vi "Actor Core.vi"(8 "error in":errorcluster, 11 "Measure Object in":refnum<class "LabJack Recorder.lvclass">) -> (0 "error out":errorcluster, 3 "Actor out":refnum<class "Actor.lvclass">)   [LabVIEW 2021, in "LabJack Recorder.lvclass"]
doc: "(<B>Filename</B>: Actor Framework.lvlib:Actor.lvclass:Actor Core.vi)\n\nReceives messages to the actor, reacts to them, and initiates any error handling that may shut the actor down.\n\nDescendant classes may override this VI to append parallel tasks for the actor to complete while it handles messages. Overrides use the Call Parent Method node."
uses:
  LabJack Recorder.lvclass
  <vilib>/ActorFramework/Actor/Actor.lvclass
  NHMFL_Core/Libraries/Instruments/LabJack/LabJack Configuration.ctl
  Continuous Recorder Actor/Continuous Recorder Actor.lvclass
panel:
  in  "Configuration":T1={"Scale"=-443.074, "Offset"=532.969, "AIN Range"=0, "Positive channel #"=0, "Negativ channel #"=15} {"AIN Range" items=["LJ_rgBIP10V", "LJ_rgBIP1V", "LJ_rgBIPP1V", "LJ_rgBIPP01V"]}
  out "Name":string
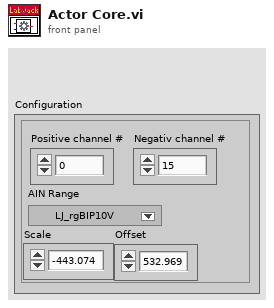
[diagram p1: front panel]
types:
  T1 = typedef "LabJack Configuration.ctl" = cluster{"Scale":dbl, "Offset":dbl, "AIN Range":u16, "Positive channel #":i32, "Negativ channel #":i32}
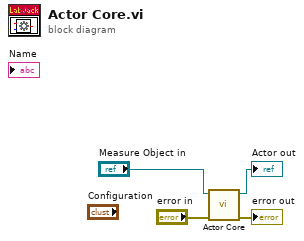
[diagram p0: block diagram]
diagram:
  n1 = call-parent "Actor Core.vi"("error in"="error in", "Measure Object in"="Measure Object in") -> ("error out"=→"error out":errorcluster, "Actor out"=→"Actor out":refnum<class "Actor.lvclass">)  [unwired: 8 in]
